vi "pb_core_clock.vi"(8 "error in (no error)":errorcluster, 10 "clock_freq (MHz)":dbl=100.0, 11 "path in":path=path "C:/Program Files/SpinCore/SpinAPI/dll/spinapi.dll") -> (0 "error out":errorcluster, 3 "path out":path)   [LabVIEW 2016]
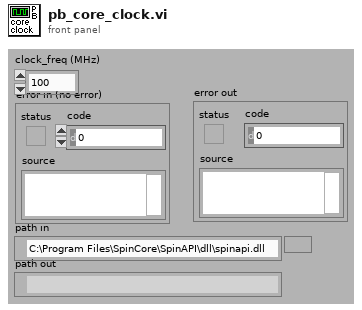
[diagram p1: front panel]
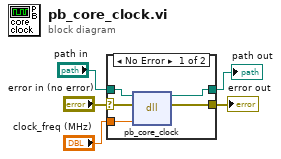
[diagram p0: block diagram]
diagram:
  n1 = case shown="No Error" "error in (no error)" {
    selector: "error in (no error)" -> [w9 w12]
    tunnel: "clock_freq (MHz)" -> [w10 _]
    tunnel: [w8 w12] -> w3
    tunnel: "path in" -> [w7 w11]
    tunnel: [w6 w11] -> w5
    frame No Error {
      n2 = dll-call lib="C:/Program Files/SpinCore/SpinAPI/dll/spinapi.dll" fn="pb_core_clock"(path in=w7, error in=w9, "clock_freq"=w10) -> (path out=w6:path, error out=w8:errorcluster)  [unwired: 2 in, 1 out]
    }
    frame Error {
    }
  }
  "error out" <- w3
  "path out" <- w5
